vi "PFI-28000-Chan-28144-I_Set Gage.vi"(8 "error in (no error)":errorcluster, 10 "Gage":T1, 11 "PFI-28000-Chan-28144-I in":refnum<class "PFI-28000-Chan-28144-I.lvclass">) -> (0 "error out":errorcluster, 3 "PFI-28000-Chan-28144-I out":refnum<class "PFI-28000-Chan-28144-I.lvclass">)   [LabVIEW 2017, in "PFI-28000-Chan-28144-I.lvclass"]
uses:
  PFI-28000-Chan-28144-I.lvclass
  C:/wc/07143 Precision Filters 28000 Support/Driver/source/Channel/PFI-28000-Channel.lvclass
  PFI-28000-Chan-28144-Gage.ctl
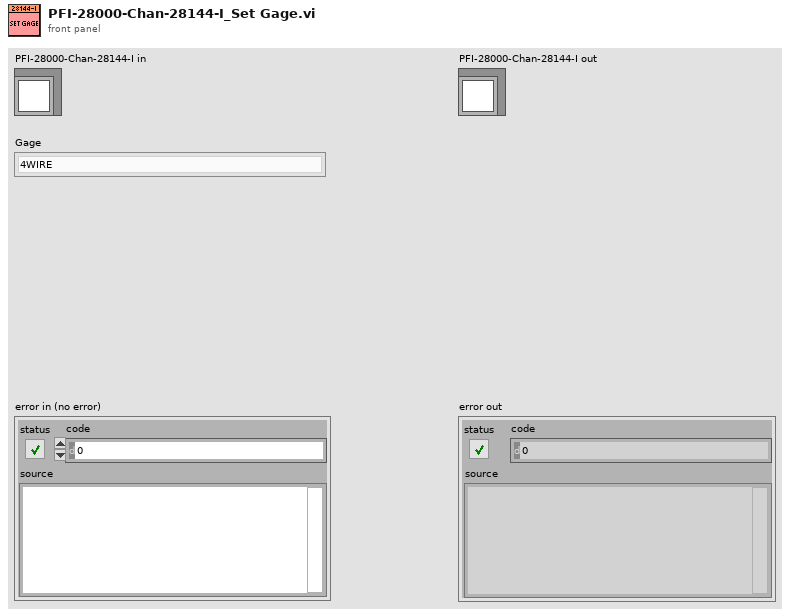
[diagram p1: front panel]
types:
  T1 = typedef "PFI-28000-Chan-28144-I.lvclass/PFI-28000-Chan-28144-Gage.ctl" = enum8{"4WIRE", "2WIRE"}
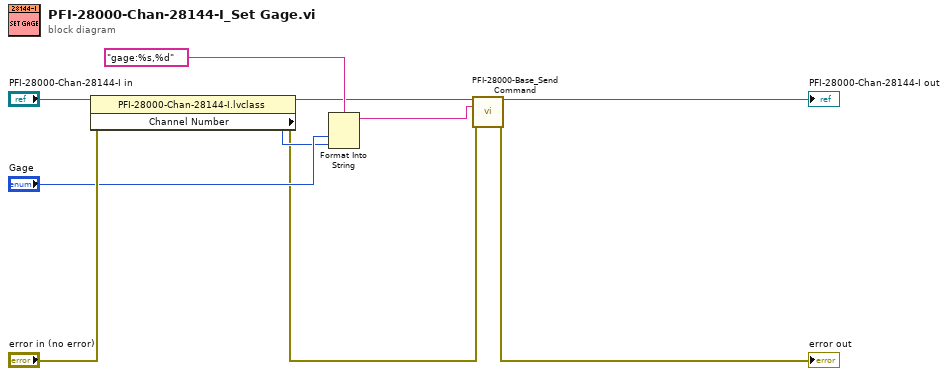
[diagram p0: block diagram]
diagram:
  n1 = property class="PFI-28000-Chan-28144-I.lvclass"(reference="PFI-28000-Chan-28144-I in", error in="error in (no error)") -> (reference out=w5:refnum<class "PFI-28000-Chan-28144-I.lvclass">, error out=w3:errorcluster, "Channel Number"=w6:i32)
  n2 = Format Into String(format string="gage:%s,%d" ("empty string"), "Gage", w6) -> (resulting string=w1:string)  [unwired: 2 in, 1 out]
  n3 = call-dynamic "PFI-28000-Base_Send Command.vi"("PFI-28000-Base in"=w5, "Command"=w1, "error in (no error)"=w3) -> ("PFI-28000-Base out"=→"PFI-28000-Chan-28144-I out":refnum<class "PFI-28000-Chan-28144-I.lvclass">, "error out"=→"error out":errorcluster)  [unwired: 11 in]
